vi "Data.Build Result Numeric.vi"(4 "Desc":string, 6 "Code":i32, 7 "Category":string, 8 "Error":errorcluster, 9 "Limit Def":T1, 10 "Value":dbl, 11 "Name":string) -> (3 "Measurement":T3 {"Status" items=["LOG", "PASS", "FAIL", "ERROR"]})   [LabVIEW 2024, in "EQMF.lvlib" / "Data.lvlib"]
uses:
  Data.lvlib
  TypeDefs/Data.Result Numeric.ctl
  TypeDefs/Data.Result Numeric Limit Type.ctl
  TypeDefs/Data.Result Item Status.ctl
  TypeDefs/Data.Result Numeric Limit Type with Limits.ctl
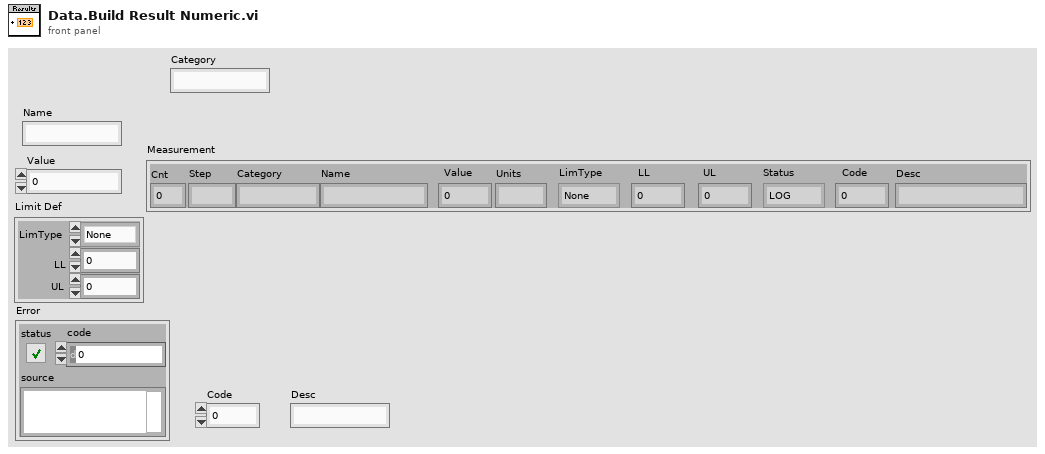
[diagram p1: front panel]
types:
  T1 = typedef "EQMF.lvlib/Data.lvlib/Data.Result Numeric Limit Type with Limits.ctl" = cluster{"LimType":T2, "LL":dbl, "UL":dbl}
  T2 = typedef "EQMF.lvlib/Data.lvlib/Data.Result Numeric Limit Type.ctl" = enum16{"None", "EQ", "NE", "GT", "LT", "GE", "LE", "GTLT", "GELE", "GELT", "GTLE", "LTGT", "LEGE", "LEGT", "LTGE"}
  T3 = typedef "EQMF.lvlib/Data.lvlib/Data.Result Numeric.ctl" = cluster{"Cnt":i32, "Step":string, "Category":string, "Name":string, "Value":dbl, "Units":string, "LimType":T2, "LL":dbl, "UL":dbl, "Status":T4, "Code":i32, "Desc":string}
  T4 = typedef "EQMF.lvlib/Data.lvlib/Data.Result Item Status.ctl" = i32
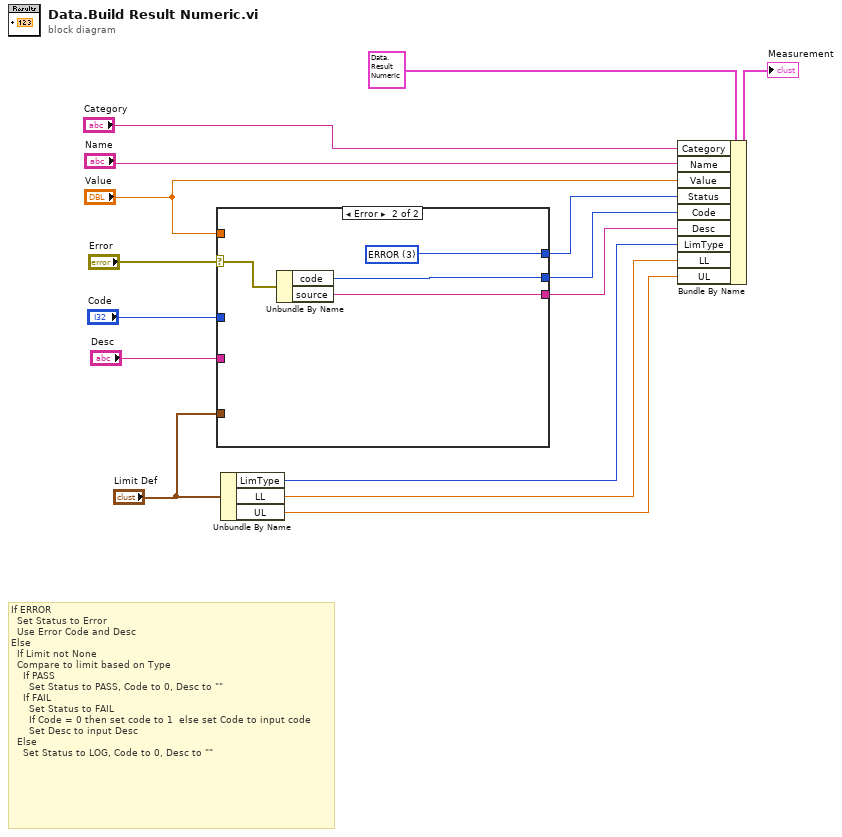
[diagram p0: block diagram]
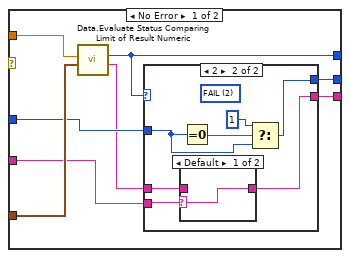
[diagram p2: hidden frame]
diagram:
  # "If ERROR\n  Set Status to Error\n  Use Error Code and Desc\nElse\n  If Limit not None\n  Compare to limit based on Type\n    If PASS\n      Set Status to PASS, Code to 0, Desc to \"\"\n    If FAIL\n      Set Status to FAIL\n      If Code = 0 then set code to 1  else set Code to input code\n      Set Desc to input Desc\n  Else\n    Set Status to LOG, Code to 0, Desc to \"\""
  n1 = case shown="Error" "Error" {
    selector: "Error" -> [_ w36]
    tunnel: "Code" -> [w20 _]
    tunnel: "Desc" -> [w19 _]
    tunnel: "Limit Def" -> [w22 _]
    tunnel: [w21 w33] -> w4
    tunnel: [w18 w35] -> w3
    tunnel: [w16 w34] -> w2
    tunnel: "Value" -> [w23 _]
    frame No Error {
      n2 = call "Data.Evaluate Status Comparing Limit of Result Numeric.vi"("Limit Def"=w22, "Value"=w23) -> ("Desc"=w17:string, "Status"=w21:T4)  [unwired: 8 in]
      n3 = case shown="2" w21 {
        tunnel: w20 -> [_ w29]
        tunnel: w19 -> [_ w26]
        tunnel: [_ w27] -> w18
        tunnel: w17 -> [_ w25]
        tunnel: [_ w24] -> w16
        frame 0, Default {
        }
        frame 2 {
          (unwired) T4 2 items=["LOG", "PASS", "FAIL", "ERROR"] ("Status")
          n4 = case shown="Default" w26 {
            selector: w26 -> [w31 _]
            tunnel: w25 -> [_ w32]
            tunnel: [w31 w32] -> w24
            frame Default {
            }
            frame "" {
            }
          }
          n5 = Equal To 0?(x=w29) -> (x = 0?=w30:bool)
          n6 = Select(t=1, s=w30, f=w29) -> (s? t:f=w27:i32)
        }
      }
    }
    frame Error {
      w33 = T4 3 items=["LOG", "PASS", "FAIL", "ERROR"] ("Status")
      n7 = Unbundle By Name(w36) -> ("code"=w35:i32, "source"=w34:string)
    }
  }
  n8 = Unbundle By Name("Limit Def") -> ("LimType"=w11:T2, "LL"=w10:dbl, "UL"=w9:dbl)
  n9 = Bundle By Name(cluster=T3 {"Cnt"=0, "Step"="", "Category"="", "Name"="", "Value"=0.0, "Units"="", "LimType"=enum."None", "LL"=0.0, "UL"=0.0, "Status"=0, "Code"=0, "Desc"=""} ("Measurement"), "Category"="Category", "Name"="Name", "Value"="Value", "Status"=w4, "Code"=w3, "Desc"=w2, "LimType"=w11, "LL"=w10, "UL"=w9) -> (→"Measurement":T3)
